vi "JTAG F-RAM Startup.vi"(8 "error in (no error)":errorcluster, 9 "Set Data":bool, 10 "Data":u8 format="%02x", 11 "Location":u16(ring)=32704 items=["STARTUP"=32704, "STIM_TRIM_FLAGS"=32705, "PWR_TRIM_FLAGS"=32706, "MICS_TRIM_FLAGS"=32707, "<undefined>"=32708, "<undefined>"=32709, "<undefined>"=32710, "<undefined>"=32711, "<undefined>"=32712, "<undefined>"=32713, "<undefined>"=32714, "<undefined>"=32715, "<undefined>"=32716, "<undefined>"=32717, "<undefined>"=32718, "<undefined>"=32719, "PWR_TRIM0"=32720, "PWR_TRIM1"=32721, "PWR_TRIM2"=32722, "PWR_TRIM3"=32723, "PWR_TRIM4"=32724, "PWR_TRIM5"=32725, "PWR_TRIM6"=32726, "PWR_TRIM7"=32727, "PWR_TRIM8"=32728, "PWR_TRIM9"=32729, "PWR_TRIM10"=32730, "PWR_<undefined>"=32731, "PWR_<undefined>"=32732, "PWR_<undefined>"=32733, "PWR_<undefined>"=32734, "PWR_<undefined>"=32735, "STIM_BG_TRIM"=32736, "STIM_CG_TRIM"=32737, "STIM_PGO_TRIM"=32738, "STIM_<undefined>"=32739, "STIM_<undefined>"=32740, "STIM_<undefined>"=32741, "STIM_<undefined>"=32742, "STIM_<undefined>"=32743, "STIM_<undefined>"=32744, "STIM_<undefined>"=32745, "STIM_<undefined>"=32746, "STIM_<undefined>"=32747, "STIM_<undefined>"=32748, "STIM_<undefined>"=32749, "STIM_<undefined>"=32750, "STIM_<undefined>"=32751, "MICS_<undefined>"=32752, "MICS_<undefined>"=32753, "MICS_<undefined>"=32754, "MICS_<undefined>"=32755, "MICS_<undefined>"=32756, "MICS_<undefined>"=32757, "MICS_<undefined>"=32758, "MICS_<undefined>"=32759, "MICS_<undefined>"=32760, "MICS_<undefined>"=32761, "MICS_<undefined>"=32762, "MICS_<undefined>"=32763, "MICS_<undefined>"=32764, "MICS_<undefined>"=32765, "MICS_<undefined>"=32766, "MICS_<undefined>"=32767]) -> (0 "error out":errorcluster, 2 "Readback":u8 format="%02x")   [LabVIEW 2009]
panel:
  # "STARTUP:\n    Bit 1: Set UV_PROT\n    Bit 2: Set LDO_CTL\n    Bit 3: Set Pluto Trims\n    Bit 4: Perform STIM Dig Startup\n    Bit 5: Perform STIM BBC Startup"
  # "STIM_TRIMS:\n    Bit 1: BG_TRIM Valid\n    Bit 2: CG_TRIM Valid\n    Bit 3: PGO_TRIM Valid"
  # "PWR_TRIMS:\n    Bit 1: Trim All From FRAM"
  # "MICS_TRIMS:\n    Bit 1: <undefined>"
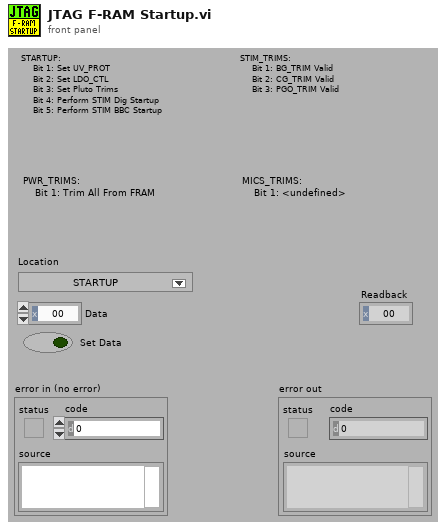
[diagram p1: front panel]
types:
  T1 = enum16{"Power UP", "Power DN", "Read Single", "Write Single", "Read Block", "Write Block", "Read SR", "Write SR", "Send Opcode"}
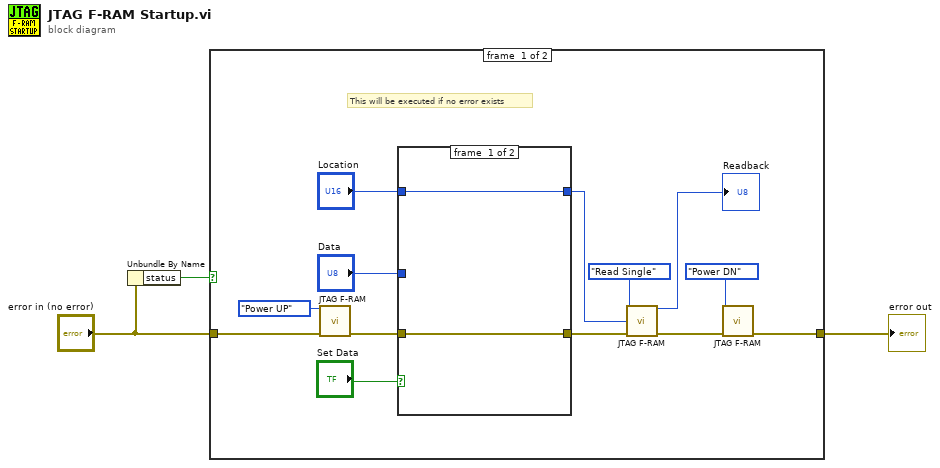
[diagram p0: block diagram]
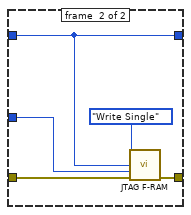
[diagram p2: hidden frame]
diagram:
  n1 = Unbundle By Name("error in (no error)") -> ("status"=w2:bool)
  n2 = case shown="False" w2 {
    tunnel: [w6 w24] -> w3
    tunnel: "error in (no error)" -> [w10 w24]
    frame #0 {
      # "This will be executed if no error exists"
      n3 = call "JTAG F-RAM.vi"("Function"=T1."Power UP", "error in (no error)"=w10) -> ("error out"=w13:errorcluster)  [unwired: 11 in, 2 out]
      n4 = case shown="True" "Set Data" {
        tunnel: w13 -> [w18 w23]
        tunnel: "Location" -> [w17 w19]
        tunnel: "Data" -> [_ w21]
        tunnel: [w18 w20] -> w11
        tunnel: [w17 w19] -> w9
        frame #0 {
        }
        frame #1 {
          n5 = call "JTAG F-RAM.vi"("Function"=T1."Write Single", "Address"=w19, "Value"=w21, "error in (no error)"=w23) -> ("error out"=w20:errorcluster)  [unwired: 9 in, 2 out]
        }
      }
      n6 = call "JTAG F-RAM.vi"("Function"=T1."Read Single", "Address"=w9, "error in (no error)"=w11) -> ("Read Value"=→"Readback":u8, "error out"=w7:errorcluster)  [unwired: 10 in, 1 out]
      n7 = call "JTAG F-RAM.vi"("Function"=T1."Power DN", "error in (no error)"=w7) -> ("error out"=w6:errorcluster)  [unwired: 11 in, 2 out]
    }
    frame #1 {
      # "Error exists, skip all functions"
    }
  }
  "error out" <- w3
